vi "Save data.vi"(8 "error in (no error)":errorcluster, 10 "data":T3, 11 "file refs":T1 {"file" format="%.0x"}) -> (0 "error out":errorcluster, 3 "file refs out":T1 {"file" format="%.0x"})   [LabVIEW 2013]
uses:
  File refs.ctl
  <vilib>/addons/h5labview2/base/hid_t.ctl
  Data.ctl
  HDF5 append data (DBL 2D).vi
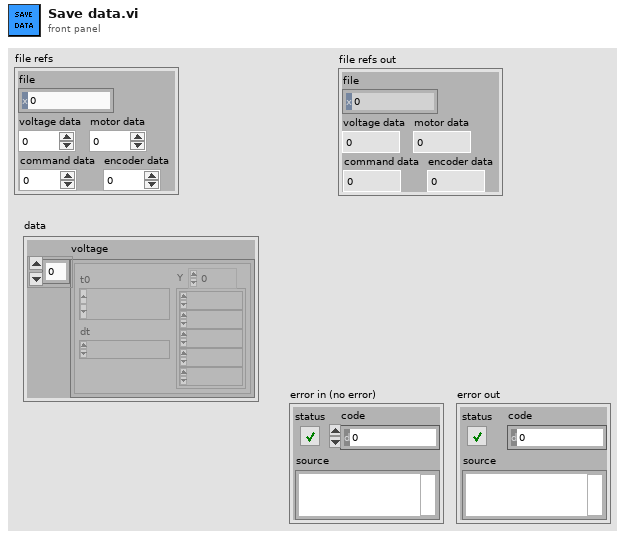
[diagram p1: front panel]
types:
  T1 = typedef "File refs.ctl" = cluster{"file":T2, "voltage data":i32, "motor data":i32, "command data":i32, "encoder data":i32}
  T2 = typedef "hid_t.ctl" = i32
  T3 = typedef "Data.ctl" = cluster{"voltage":waveform(dbl)[]}
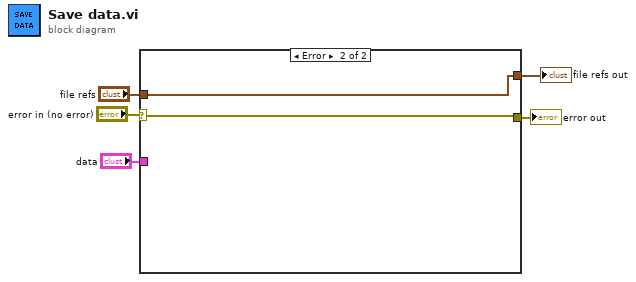
[diagram p0: block diagram]
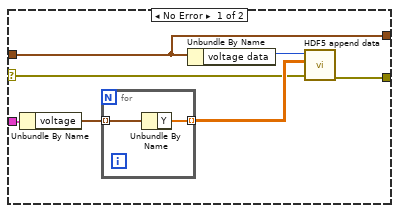
[diagram p2: hidden frame]
diagram:
  n1 = case shown="Error" "error in (no error)" {
    selector: "error in (no error)" -> [w7 w16]
    tunnel: "file refs" -> [w6 w15]
    tunnel: "data" -> [w11 _]
    tunnel: [w8 w16] -> w3
    tunnel: [w6 w15] -> w1
    frame No Error {
      n2 = Unbundle By Name(w11) -> ("voltage"=w10:waveform(dbl)[])
      n3 = for {
        tunnel: w10 -> [w14] mode=indexing
        tunnel: [w13] -> w9 mode=indexing
        n4 = Unbundle By Name(w14) -> ("Y"=w13:dbl[])
      }
      n5 = Unbundle By Name(w6) -> ("voltage data"=w12:i32)
      n6 = call-poly "HDF5 append data.vi"("error in (no error)"=w7, "data"=w9, "dset in"=w12) -> ("error out"=w8:errorcluster)  [unwired: 7 in, 1 out]
    }
    frame Error {
    }
  }
  "error out" <- w3
  "file refs out" <- w1
